vi "Initialize_MacroGen_MD.vi"(8 "Error In":errorcluster, 11 "UI control refnums":T1) -> (0 "Error Out":errorcluster)   [LabVIEW 2012]
uses:
  Custom Controls and Typedefs/Macro_MD_UI Control Refnums.ctl
  Custom Controls and Typedefs/Delete Button.ctl
  Custom Controls and Typedefs/Edit Button.ctl
  FGV_MacroGen_Commands.ctl
  <vilib>/Utility/miscctls.llb/LVRowAndColumnTypeDef.ctl
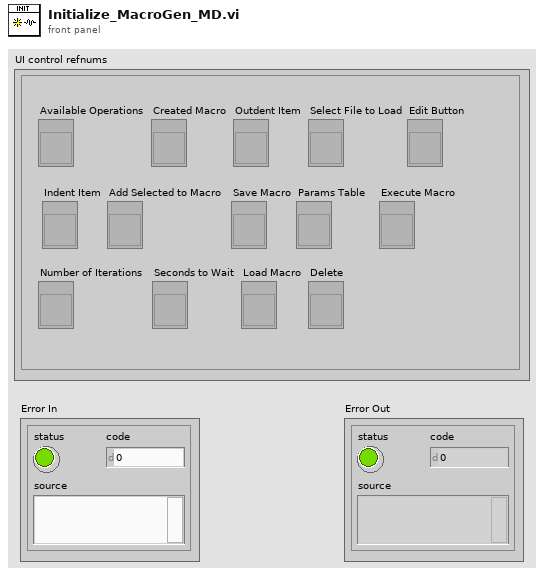
[diagram p1: front panel]
types:
  T1 = typedef "Macro_MD_UI Control Refnums.ctl" = cluster{"Available Operations":refnum<vi>, "Created Macro":refnum<vi>, "Indent Item":refnum<vi>, "Add Selected to Macro":refnum<vi>, "Outdent Item":refnum<vi>, "Number of Iterations":refnum<vi>, "Seconds to Wait":refnum<vi>, "Load Macro":refnum<vi>, "Save Macro":refnum<vi>, "Select File to Load":refnum<vi>, "Params Table":refnum<vi>, "Delete":refnum<vi>, "Edit Button":refnum<vi>, "Execute Macro":refnum<vi>}
  T2 = typedef "FGV_MacroGen_Commands.ctl" = enum16{"Initialize", "Get Array", "Load from file", "Insert Item", "Insert at End", "Edit Item", "Delete Item", "Move Items", "Save", "SaveAs"}
  T3 = typedef "LVRowAndColumnTypeDef.ctl" = cluster{"Row":i32, "Column":i32}
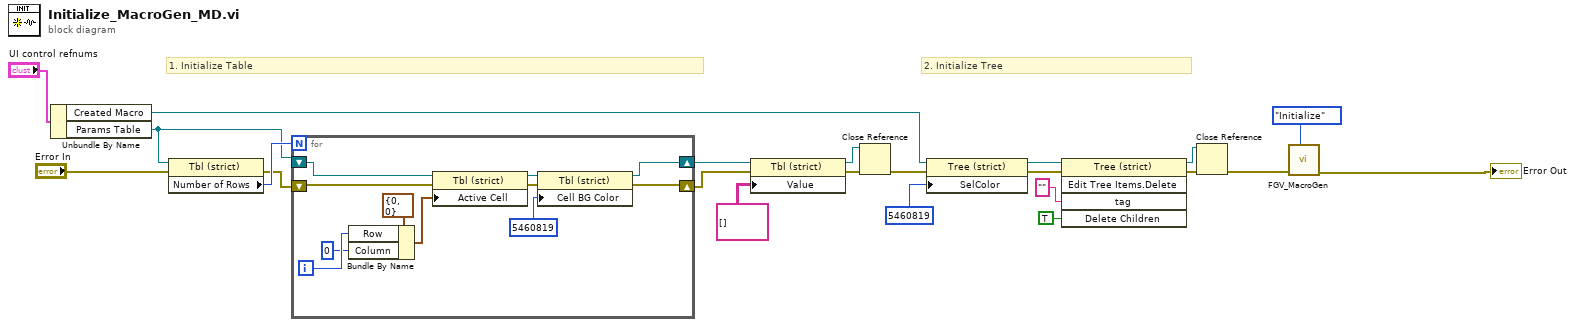
[diagram p0: block diagram]
diagram:
  # "2. Initialize Tree"
  # "1. Initialize Table"
  n1 = Unbundle By Name("UI control refnums") -> ("Created Macro"=w13:refnum<vi>, "Params Table"=w20:refnum<vi>)
  n2 = property class="Tbl (strict)"(reference=w20, error in="Error In") -> (error out=w18:errorcluster, "Number of Rows"=w21:u32)  [unwired: 1 out]
  n3 = for {
    N: w21 -> [_]
    shift-right: [w25] -> w4
    shift-left: w18 -> [w26]
    shift-right: [w24] -> w5
    shift-left: w20 -> [w29]
    i -> [w32]
    n4 = Bundle By Name(cluster=T3 {"Row"=0, "Column"=0} ("Active Cell:Active Cell"), "Row"=w32, "Column"=0) -> (w30:T3)
    n5 = property class="Tbl (strict)"(reference=w29, error in=w26, "Active Cell"=w30) -> (reference out=w27:refnum<vi>, error out=w28:errorcluster)
    n6 = property class="Tbl (strict)"(reference=w27, error in=w28, "Cell BG Color"=u32 5460819 ("Active Cell:Cell Background Color")) -> (reference out=w24:refnum<vi>, error out=w25:errorcluster)
  }
  n7 = property class="Tbl (strict)"(reference=w5, error in=w4, "Value"=string[][] []) -> (reference out=w7:refnum<vi>, error out=w6:errorcluster)
  n8 = Close Reference(reference=w7, error in (no error)=w6) -> (error out=w3:errorcluster)
  n9 = property class="Tree (strict)"(reference=w13, error in=w3, "SelColor"=u32 5460819 ("Active Cell:Cell Background Color")) -> (reference out=w14:refnum<vi>, error out=w15:errorcluster)
  n10 = invoke class="Tree (strict)" method="Edit Tree Items.Delete"(reference=w14, error in=w15, "tag"="" ("Tag"), "Delete Children"=TRUE ("Delete Children?")) -> (reference out=w11:refnum<vi>, error out=w12:errorcluster)  [unwired: 1 in, 3 out]
  n11 = Close Reference(reference=w11, error in (no error)=w12) -> (error out=w9:errorcluster)
  n12 = call "FGV_MacroGen.vi"("MacroFGV_Commands"=FGV_MacroGen_Commands."Initialize", "Error In"=w9) -> ("Error Out"=→"Error Out":errorcluster)  [unwired: 7 in, 2 out]
